vi "init 12V power supply.vi"(8 "error in":errorcluster, 11 "VISA Refnum in":refnum<visa-resource-name>) -> (0 "error out":errorcluster)   [LabVIEW 2020]
uses:
  Hardware Drivers/Keysight E3633 DC PS/dc ps control.ctl
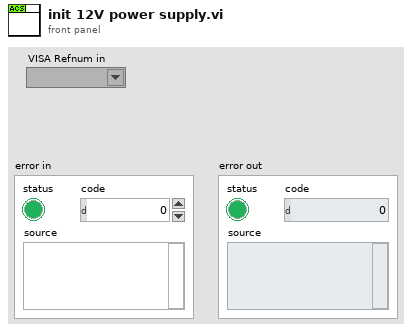
[diagram p1: front panel]
types:
  T1 = typedef "dc ps control.ctl" = enum16{"init", "config output", "config OVP", "config current limit", "output on_off", "read output", "self test", "close"}
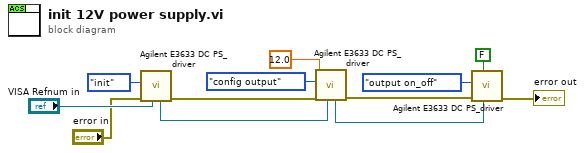
[diagram p0: block diagram]
diagram:
  n1 = call "Agilent E3633 DC PS_driver.vi"("VISA resource in"="VISA Refnum in", "Error In"="error in", "agilent E3633 DC PS"=dc_ps_control."init") -> ("Error Out"=w11:errorcluster, "VISA resource name out"=w7:refnum<visa-resource-name>)  [unwired: 5 in, 2 out]
  n2 = call "Agilent E3633 DC PS_driver.vi"("VISA resource in"=w7, "Error In"=w11, "value in"=12.0, "agilent E3633 DC PS"=dc_ps_control."config output") -> ("Error Out"=w12:errorcluster, "VISA resource name out"=w9:refnum<visa-resource-name>)  [unwired: 4 in, 2 out]
  n3 = call "Agilent E3633 DC PS_driver.vi"("VISA resource in"=w9, "Enable Output (T: Enable)"=FALSE, "Error In"=w12, "agilent E3633 DC PS"=dc_ps_control."output on_off") -> ("Error Out"=→"error out":errorcluster)  [unwired: 4 in, 3 out]
